vi "VI Ref FGV.vi"(7 "FGV CMD":T1, 8 "error in (no error)":errorcluster, 11 "VI Ref":refnum<vi>[](array[refnum])) -> (0 "error out":errorcluster, 3 "VI Ref 2":refnum<vi>[](array[refnum]))   [LabVIEW 2021]
uses:
  Controls/FGV CMD.ctl
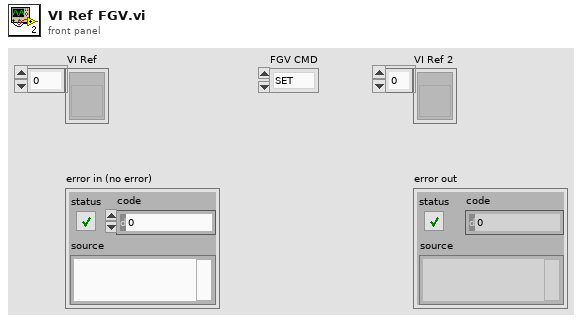
[diagram p1: front panel]
types:
  T1 = typedef "FGV CMD.ctl" = enum16{"SET", "GET", "CLEAR"}
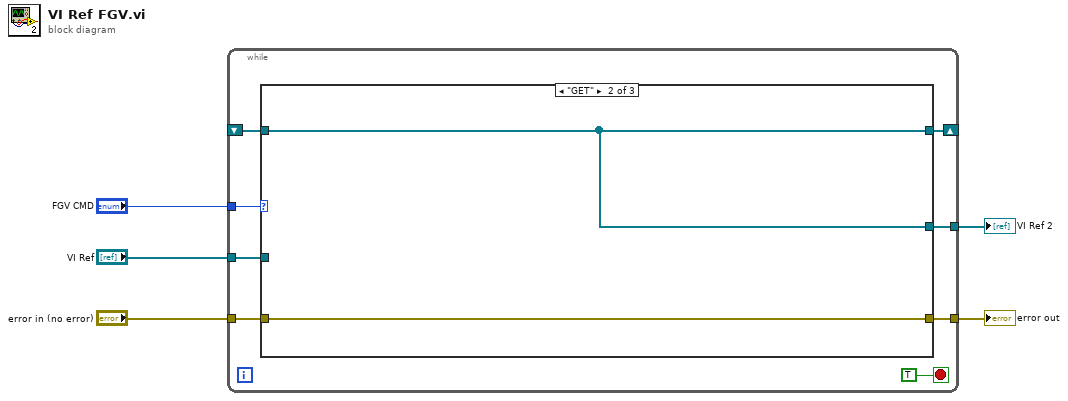
[diagram p0: block diagram]
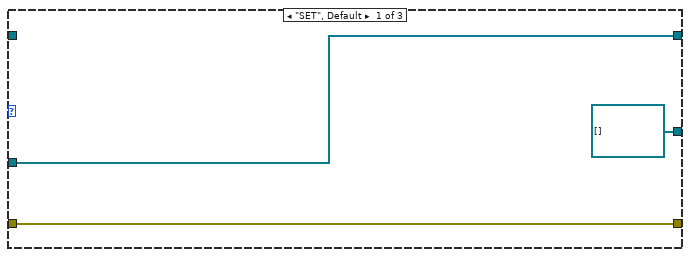
[diagram p2: hidden frame]
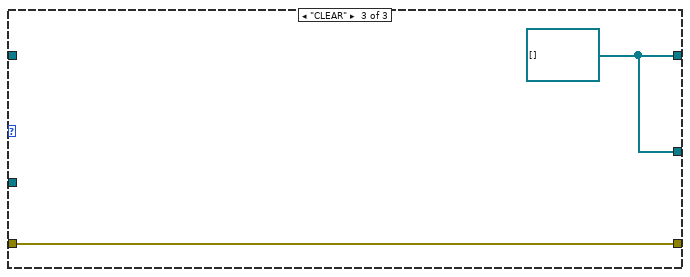
[diagram p3: hidden frame]
diagram:
  n1 = while {
    shift-right: [w10] -> _
    shift-left: _ -> [w8]
    tunnel: "FGV CMD" -> [w13]
    tunnel: "VI Ref" -> [w11]
    tunnel: [w9] -> w3
    tunnel: "error in (no error)" -> [w7]
    tunnel: [w6] -> w1
    stop <- TRUE stop-if-true
    n2 = case shown="\"GET\"" w13 {
      tunnel: w11 -> [w16 _ _]
      tunnel: [w16 w18 w20] -> w10
      tunnel: w8 -> [_ w18 _]
      tunnel: [refnum<vi>[] [] ("VI Ref") w18 w20] -> w9
      tunnel: w7 -> [w14 w17 w19]
      tunnel: [w14 w17 w19] -> w6
      frame "SET", Default {
      }
      frame "GET" {
      }
      frame "CLEAR" {
        w20 = refnum<vi>[] [] ("VI Ref")
      }
    }
  }
  "VI Ref 2" <- w3
  "error out" <- w1
